vi "Read Trigger Type.vi"(8 "error in (no error)":errorcluster, 11 "Trigger in":refnum<class "Trigger.lvclass">) -> (0 "error out":errorcluster, 2 "Trigger Type":T1, 3 "Trigger out":refnum<class "Trigger.lvclass">)   [LabVIEW 2012, in "Waveform Data Logger Engine.lvlib" / "Trigger.lvclass"]
uses:
  Trigger.lvclass
  Trigger Type.ctl
  Trigger.lvclass/Trigger.ctl
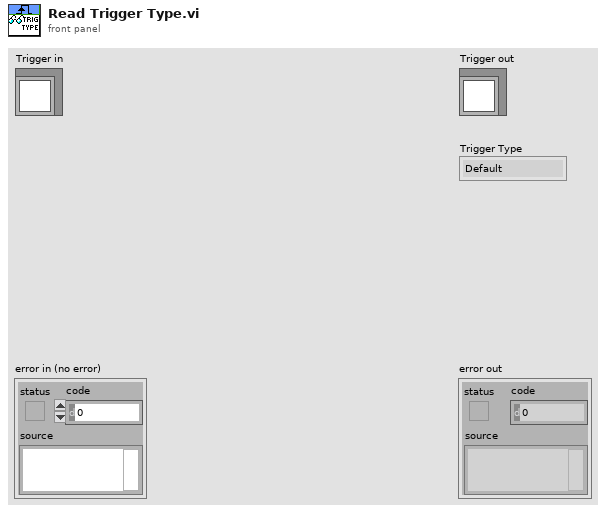
[diagram p1: front panel]
types:
  T1 = typedef "Waveform Data Logger Engine.lvlib/Trigger.lvclass/Trigger Type.ctl" = enum16{"Default", "Digital Edge", "Analog Edge", "In Range", "Value Change", "Boolean Evaluation"}
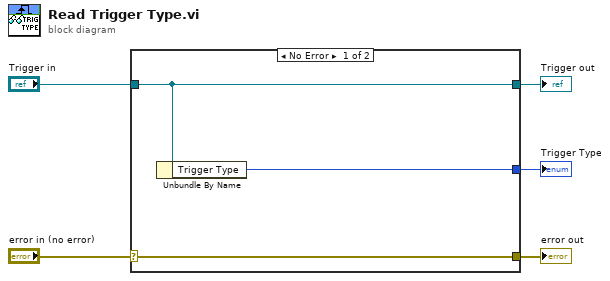
[diagram p0: block diagram]
diagram:
  n1 = case shown="No Error" "error in (no error)" {
    selector: "error in (no error)" -> [w8 w9]
    tunnel: [w8 w9] -> w4
    tunnel: [w7 w10] -> w2
    tunnel: "Trigger in" -> [w7 w10]
    tunnel: [w6 _] -> w1
    frame No Error {
      n2 = Unbundle By Name(w7) -> ("Trigger Type"=w6:T1)
    }
    frame Error {
    }
  }
  "error out" <- w4
  "Trigger out" <- w2
  "Trigger Type" <- w1
